vi "Adquisition tension.vi"(3 "Tension":dbl(slide) scale=2.0..4.0) -> (1 "Température":dbl)   [LabVIEW 2022 SP3]
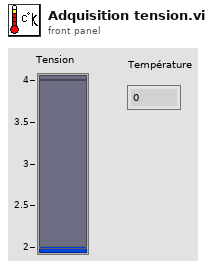
[diagram p1: front panel]
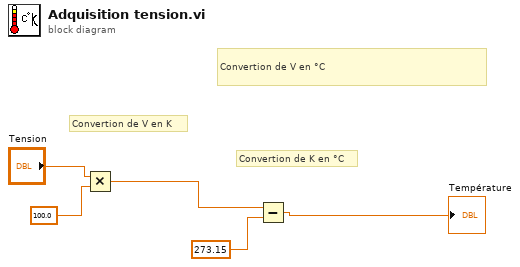
[diagram p0: block diagram]
diagram:
  # "Convertion de V en °C"
  # "Convertion de K en °C"
  # "Convertion de V en K"
  n1 = Multiply(x="Tension", y=100.0) -> (x*y=w3:dbl)
  n2 = Subtract(x=w3, y=273.15) -> (x-y=→"Température":dbl)
